vi "Select DBL Signals.vi"(8 "error in (no error)":errorcluster, 10 "Selector Input":bool[](array[boolean]), 11 "All Signals":dbl[][](array[numeric])) -> (0 "error out":errorcluster, 3 "Selected Signals":dbl[][](array[numeric]))   [LabVIEW 2013]
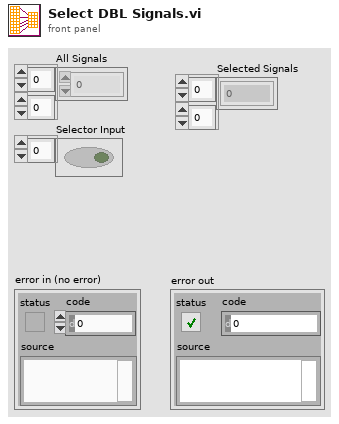
[diagram p1: front panel]
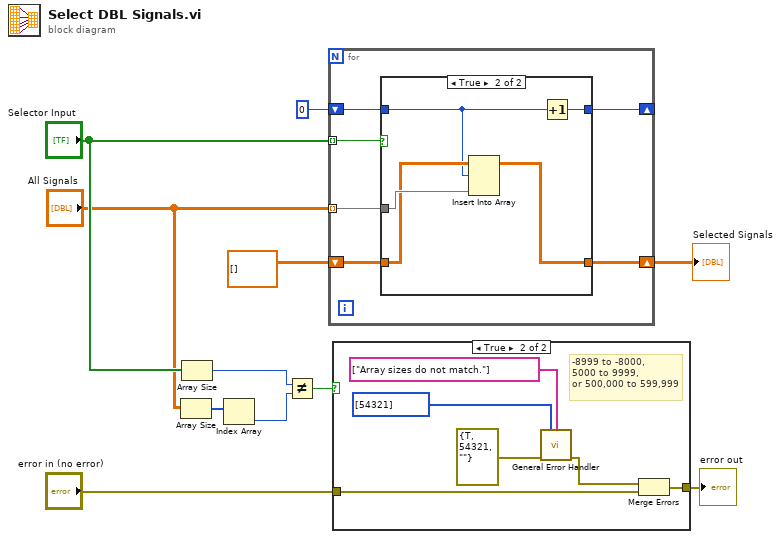
[diagram p0: block diagram]
diagram:
  n1 = Array Size(array="All Signals") -> (size(s)=w6:i32[])
  n2 = Array Size(array="Selector Input") -> (size(s)=w5:i32)
  n3 = Index Array(array=w6) -> (element=w4:i32)  [unwired: 1 in]
  n4 = Not Equal?(x=w5, y=w4) -> (x != y?=w3:bool)
  n5 = for {
    tunnel: "All Signals" -> [w16] mode=indexing
    tunnel: "Selector Input" -> [w17] mode=indexing
    shift-right: [w13] -> w9
    shift-left: dbl[][] [] ("Array") -> [w15]
    shift-right: [w12] -> _
    shift-left: 0 -> [w14]
    n6 = case shown="True" w17 {
      tunnel: w16 -> [_ w24]
      tunnel: w15 -> [w19 w23]
      tunnel: w14 -> [w18 w21]
      tunnel: [w19 w22] -> w13
      tunnel: [w18 w20] -> w12
      frame False {
      }
      frame True {
        n7 = Insert Into Array(array=w23, index (row)=w21, new element=w24) -> (w22:dbl[][])  [unwired: 1 in]
        n8 = Increment(x=w21) -> (x+1=w20:i32)
      }
    }
  }
  "Selected Signals" <- w9
  n9 = case shown="True" w3 {
    tunnel: "error in (no error)" -> [w25 w27]
    tunnel: [w25 w28] -> w1
    frame False {
    }
    frame True {
      # "-8999 to -8000,\n5000 to 9999,\nor 500,000 to 599,999"
      n10 = call <vilib>:"General Error Handler.vi"("[user-defined codes]"=i32[] [54321], "[user-defined descriptions]"=string[] ["Array sizes do not match."], "error in (no error)"=errorcluster {"status"=TRUE, "code"=54321, "source"=""}) -> ("error out"=w26:errorcluster)  [unwired: 8 in, 4 out]
      n11 = Merge Errors(w26, w27) -> (w28:errorcluster)
    }
  }
  "error out" <- w1
